vi "Start Build.vi"(0 "Open Directory?":bool, 1 "Build Package?":bool, 2 "Progres Bar":refnum<vi>, 5 "Feed":T2(ring), 7 "Feed Path":path, 9 "Selected Measurements":T1[](array[typedef]), 11 "error in (no error)":errorcluster, 12 "Package Spec":string[][](array[string])) -> (4 "Status":string[](array[string]), 15 "error out":errorcluster)   [LabVIEW 2021, in "Packager Helpers.lvlib"]
uses:
  Packager Helpers.lvlib
  controls/Build Spec Details.ctl
  <vilib>/AppBuilder/AB_API_Simple/Set Build Specification Version (path).vi
  <vilib>/AppBuilder/AB_API_Simple/Build (path).vi
  Dictionary/Dictionary.lvlib
  <vilib>/AppBuilder/AB_API_Simple/NI_App_Builder_API.lvlib
  Path Functions/Path Functions.lvlib
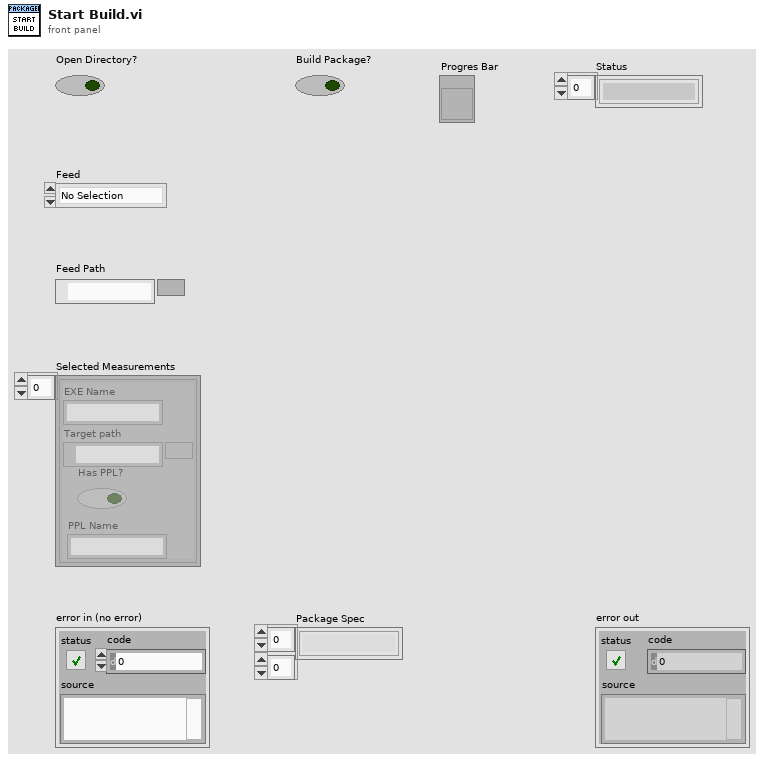
[diagram p1: front panel]
types:
  T1 = typedef "Packager Helpers.lvlib/Build Spec Details.ctl" = cluster{"EXE Name":string, "Target path":path, "Has PPL?":bool, "PPL Name":string}
  T2 = enum32{"No Selection", "CreateFeed", "AddtoFeed"}
  T3 = typedef "NI_App_Builder_API.lvlib/Build Specification Version.ctl" = cluster{"Major":u16, "Minor":u16, "Fix":u16, "Build":u16}
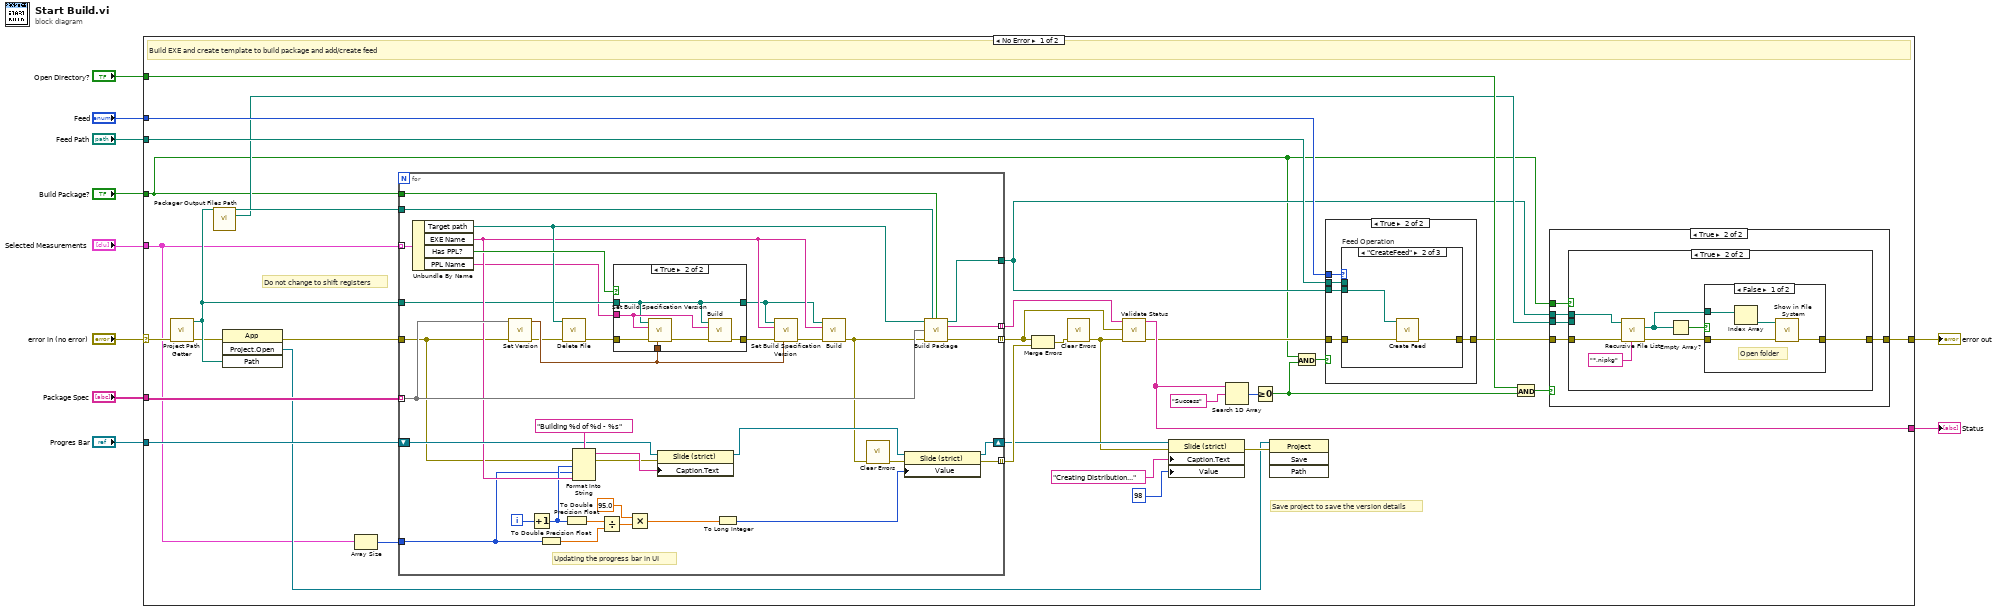
[diagram p0: block diagram]
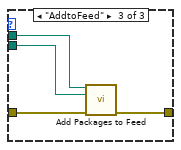
[diagram p4: hidden frame]
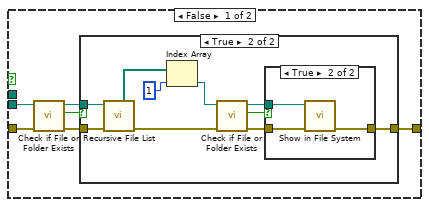
[diagram p7: hidden frame]
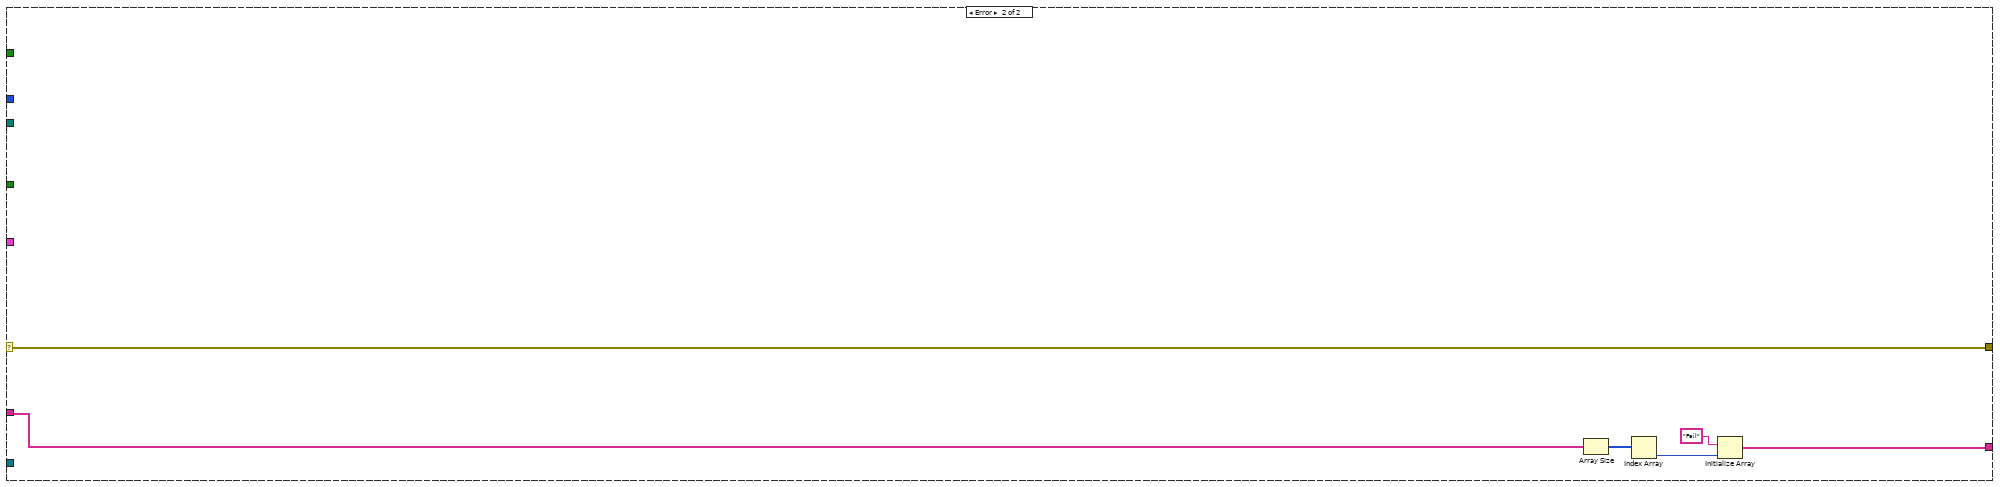
[diagram p11: hidden frame]
diagram:
  n1 = case shown="No Error" "error in (no error)" {
    selector: "error in (no error)" -> [w31 w143]
    tunnel: "Package Spec" -> [w44 w148]
    tunnel: [w38 w145] -> w9
    tunnel: "Progres Bar" -> [w29 _]
    tunnel: "Open Directory?" -> [w35 _]
    tunnel: "Feed" -> [w40 _]
    tunnel: "Feed Path" -> [w39 _]
    tunnel: "Build Package?" -> [w11 _]
    tunnel: "Selected Measurements" -> [w22 _]
    tunnel: [w16 w143] -> w10
    frame No Error {
      # "Do not change to shift registers"
      # "Save project to save the version details"
      # "Build EXE and create template to build package and add/create feed"
      n2 = call "Project Path Getter.vi"("error in (no error)"=w31) -> ("Path"=w33:path, "error out"=w30:errorcluster)  [unwired: 13 in]
      n3 = call "Packager Output Files Path.vi"("Project Path"=w33) -> ("Package Path"=w34:path, "Build Outputs Path"=w32:path)  [unwired: 13 in]
      n4 = invoke class="App" method="Project.Open"(error in=w30, "Path"=w33) -> (error out=w14:errorcluster, "Project:Open"=w23:refnum<vi>)  [unwired: 2 in, 2 out]
      n5 = Array Size(array=w22) -> (size(s)=w42:i32)
      n6 = for {
        tunnel: w14 -> [w70]
        tunnel: w22 -> [w95] mode=indexing
        tunnel: w11 -> [w85]
        tunnel: w44 -> [w78] mode=indexing
        tunnel: [w94] -> w19
        tunnel: [w63] -> w27 mode=indexing
        tunnel: [w93] -> w43 mode=indexing
        tunnel: w42 -> [w60]
        tunnel: [w82] -> w41 mode=indexing
        shift-right: [w80] -> w26
        shift-left: w29 -> [w91]
        tunnel: w33 -> [w73]
        tunnel: w34 -> [w76]
        i -> [w59]
        # "Updating the progress bar in UI"
        n7 = Unbundle By Name(w95) -> ("Target path"=w77:path, "EXE Name"=w74:string, "Has PPL?"=w79:bool, "PPL Name"=w72:string)
        n8 = call "Set Version.vi"("Package Spec"=w78, "error in (no error)"=w70) -> ("Build Specification Version"=w71:T3, "error out"=w69:errorcluster)  [unwired: 12 in]
        n9 = Increment(x=w59) -> (x+1=w61:i32)
        n10 = To Double Precision Float(number=w60) -> (double precision float=w84:dbl)
        n11 = call "Delete File.vi"("File or Folder Path"=w77, "error in (no error)"=w69) -> ("error out"=w68:errorcluster)  [unwired: 13 in]
        n12 = To Double Precision Float(number=w61) -> (double precision float=w86:dbl)
        n13 = Format Into String(format string="Building %d of %d - %s", error in=w70, w61, w60, w74) -> (resulting string=w90:string, error out=w62:errorcluster)  [unwired: 1 in]
        n14 = Divide(x=w86, y=w84) -> (x/y=w89:dbl)
        n15 = case shown="True" w79 {
          tunnel: w73 -> [w96 w98]
          tunnel: w71 -> [_ w103]
          tunnel: w72 -> [_ w102]
          tunnel: w68 -> [w97 w101]
          tunnel: [w97 w99] -> w67
          tunnel: [w96 w98] -> w66
          frame False {
          }
          frame True {
            n16 = call-poly <vilib>:"Set Build Specification Version.vi"("Build Specification Version"=w103, "error in (no error)"=w101, "Name of build specification"=w102, "Path to project"=w98) -> ("error out"=w100:errorcluster)  [unwired: 7 in]
            n17 = call-poly <vilib>:"Build.vi"("error in (no error)"=w100, "Name of build specification (if empty: build all)"=w102, "Path to project"=w98) -> ("error out"=w99:errorcluster)  [unwired: 7 in, 1 out]
          }
        }
        n18 = Multiply(x=95.0 ("y"), y=w89) -> (x*y=w87:dbl)
        n19 = property class="Slide (strict)"(reference=w91, error in=w62, "Caption.Text"=w90) -> (reference out=w75:refnum<vi>)  [unwired: 1 out]
        n20 = To Long Integer(number=w87) -> (32bit integer=w81:i32)
        n21 = call-poly <vilib>:"Set Build Specification Version.vi"("Build Specification Version"=w71, "error in (no error)"=w67, "Name of build specification"=w74, "Path to project"=w66) -> ("error out"=w65:errorcluster)  [unwired: 7 in]
        n22 = call-poly <vilib>:"Build.vi"("error in (no error)"=w65, "Name of build specification (if empty: build all)"=w74, "Path to project"=w66) -> ("error out"=w64:errorcluster)  [unwired: 7 in, 1 out]
        n23 = call <vilib>:"Clear Errors.vi"("error in (no error)"=w64) -> ("error out"=w83:errorcluster)  [unwired: 5 in, 1 out]
        n24 = property class="Slide (strict)"(reference=w75, error in=w83, "Value"=w81) -> (reference out=w80:refnum<vi>, error out=w82:errorcluster)
        n25 = call "Build Package.vi"("Destination Path"=w77, "Package Path"=w76, "Build Package?"=w85, "Package Spec"=w78, "error in (no error)"=w64) -> ("Package Directory"=w94:path, "Error Message"=w93:string, "error out"=w63:errorcluster)  [unwired: 8 in]
      }
      n26 = Merge Errors(w27, w41) -> (w28:errorcluster)
      n27 = call <vilib>:"Clear Errors.vi"("error in (no error)"=w28) -> ("error out"=w25:errorcluster)  [unwired: 5 in, 1 out]
      n28 = call "Validate Status.vi"("Error Msg[]"=w43, "Error[]"=w27, "error in (no error)"=w25) -> ("Status"=w38:string[], "error out"=w18:errorcluster)  [unwired: 11 in]
      n29 = property class="Slide (strict)"(reference=w26, error in=w25, "Caption.Text"="Creating Distribution...", "Value"=98) -> (error out=w24:errorcluster)  [unwired: 1 out]
      n30 = Search 1D Array(1D array=w38, element="Success") -> (index of element=w36:i32)  [unwired: 1 in]
      n31 = Greater Or Equal To 0?(x=w36) -> (x >= 0?=w13:bool)
      n32 = invoke class="Project" method="Save"(reference=w23, error in=w24) -> ()  [unwired: 2 in, 4 out]
      n33 = And(x=w11, y=w13) -> (x .and. y?=w12:bool)
      n34 = case shown="True" w12 {
        tunnel: w40 -> [_ w50]
        tunnel: w39 -> [_ w49]
        tunnel: w19 -> [_ w48]
        tunnel: w18 -> [w45 w47]
        tunnel: [w45 w46] -> w17
        frame False {
        }
        frame True {
          n35 = case "Feed Operation" shown="\"CreateFeed\"" w50 {
            tunnel: w49 -> [_ _ w58]
            tunnel: w48 -> [_ w54 w57]
            tunnel: w47 -> [w51 w53 w56]
            tunnel: [w51 w52 w55] -> w46
            frame "No Selection" {
            }
            frame "CreateFeed" {
              n36 = call "Create Feed.vi"("Packages Path"=w54, "error in (no error)"=w53) -> ("error out"=w52:errorcluster)  [unwired: 13 in]
            }
            frame "AddtoFeed" {
              n37 = call "Add Packages to Feed.vi"("Feed Path"=w58, "Packages Path"=w57, "error in (no error)"=w56) -> ("error out"=w55:errorcluster)  [unwired: 12 in]
            }
          }
        }
      }
      n38 = And(x=w35, y=w13) -> (x .and. y?=w15:bool)
      n39 = case shown="True" w15 {
        tunnel: w19 -> [_ w109]
        tunnel: w32 -> [_ w108]
        tunnel: [w104 w106] -> w16
        tunnel: w17 -> [w104 w107]
        tunnel: w11 -> [_ w105]
        frame False {
        }
        frame True {
          n40 = case shown="True" w105 {
            tunnel: w109 -> [_ w137]
            tunnel: w108 -> [w114 _]
            tunnel: w107 -> [w113 w136]
            tunnel: [w111 w132] -> w106
            frame False {
              n41 = call <vilib>:"Check if File or Folder Exists.vi"("error in (no error)"=w113, "path"=w114) -> ("error out"=w112:errorcluster, "file or folder exists?"=w115:bool, "dup path"=w110:path)  [unwired: 7 in]
              n42 = case shown="True" w115 {
                tunnel: w112 -> [w116 w123]
                tunnel: [w116 w118] -> w111
                tunnel: w110 -> [_ w117]
                frame False {
                }
                frame True {
                  n43 = call <vilib>:"Recursive File List.vi"("error in (no error)"=w123, "Folder Path"=w117) -> ("error out"=w121:errorcluster, "All Folders"=w126:path[])  [unwired: 5 in, 3 out]
                  n44 = Index Array(array=w126, index=1) -> (element=w125:path)
                  n45 = call <vilib>:"Check if File or Folder Exists.vi"("error in (no error)"=w121, "path"=w125) -> ("error out"=w124:errorcluster, "file or folder exists?"=w120:bool, "dup path"=w119:path)  [unwired: 7 in]
                  n46 = case shown="True" w120 {
                    tunnel: w124 -> [w127 w129]
                    tunnel: w119 -> [_ w130]
                    tunnel: [w127 w128] -> w118
                    frame False {
                    }
                    frame True {
                      n47 = call <vilib>:"Show in File System.vi"("error in (no error)"=w129, "file or directory path"=w130) -> ("error out"=w128:errorcluster)  [unwired: 9 in]
                    }
                  }
                }
              }
            }
            frame True {
              n48 = call <vilib>:"Recursive File List.vi"("pattern"="*.nipkg", "error in (no error)"=w136, "Folder Path"=w137) -> ("error out"=w133:errorcluster, "All Files in Dir"=w135:path[])  [unwired: 4 in, 3 out]
              n49 = Empty Array?(array=w135) -> (empty?=w134:bool)
              n50 = case shown="False" w134 {
                tunnel: w133 -> [w139 w142]
                tunnel: w135 -> [w141 _]
                tunnel: [w138 w142] -> w132
                frame False {
                  # "Open folder"
                  n51 = Index Array(array=w141) -> (element=w140:path)  [unwired: 1 in]
                  n52 = call <vilib>:"Show in File System.vi"("error in (no error)"=w139, "file or directory path"=w140) -> ("error out"=w138:errorcluster)  [unwired: 9 in]
                }
                frame True {
                }
              }
            }
          }
        }
      }
    }
    frame Error {
      n53 = Array Size(array=w148) -> (size(s)=w147:i32[])
      n54 = Index Array(array=w147) -> (element=w146:i32)  [unwired: 1 in]
      n55 = Initialize Array("Fail", w146) -> (w145:string[])
    }
  }
  "error out" <- w10
  "Status" <- w9
